vi "cmd2.vi"(6 "String":string) -> (0 "error out":errorcluster, 2 "String 2":string)   [LabVIEW 2010]
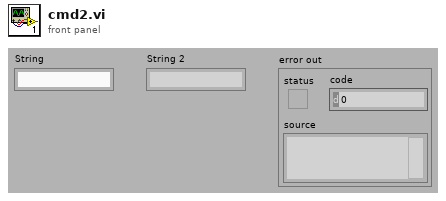
[diagram p1: front panel]
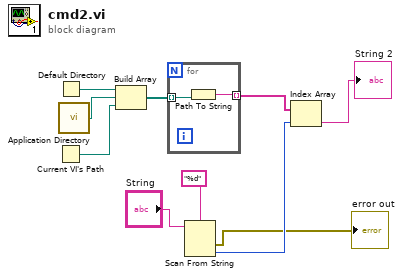
[diagram p0: block diagram]
diagram:
  n1 = Default Directory() -> (w10:path)
  n2 = Current VI's Path() -> (path=w8:path)
  n3 = call <vilib>:"Application Directory.vi"() -> ("Application Directory"=w9:path)
  n4 = Build Array(w10, w9, w8) -> (w7:path[])
  n5 = for {
    tunnel: w7 -> [w12] mode=indexing
    tunnel: [w11] -> w3 mode=indexing
    n6 = Path To String(path=w12) -> (string=w11:string)
  }
  n7 = Scan From String(format string="%d", input string="String") -> (error out=→"error out":errorcluster, output 1=w4:i32)  [unwired: 3 in, 2 out]
  n8 = Index Array(array=w3, index=w4) -> (element=→"String 2":string)
